vi "Calibration_CreateFromMatrix.vi"(1 "sample points":cluster{dbl, dbl}[](array[cluster])=[{0.0, 0.0}, {1.0, 0.0}, {0.0, 1.0}], 2 "Linear conversion Matrix":dbl[][](array[numeric])=[[1.0, 0.0, 0.0], [0.0, 1.0, 0.0]]) -> (0 "CalibrationCoordinates: x,x',y,y'...":dbl[][](array[numeric])=[[0.0, 0.0, 0.0, 0.0], [1.0, 1.0, 0.0, 0.0], [0.0, 0.0, 1.0, 1.0]])   [LabVIEW 2011]
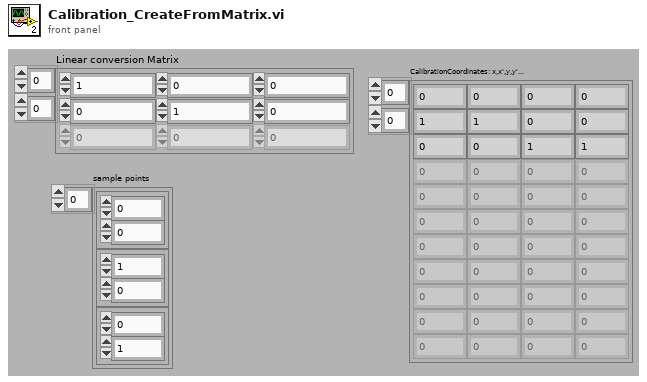
[diagram p1: front panel]
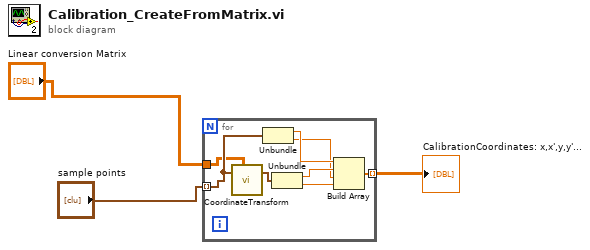
[diagram p0: block diagram]
diagram:
  n1 = for {
    tunnel: "Linear conversion Matrix" -> [w4]
    tunnel: "sample points" -> [w6] mode=indexing
    tunnel: [w11] -> w2 mode=indexing
    n2 = call "CoordinateTransform.vi"("input coordiantes"=w6, "Conversion Matrix"=w4) -> ("output coordiantes"=w5:cluster{"x":dbl, "y":dbl})  [unwired: 2 in, 1 out]
    n3 = Unbundle(w6) -> (w10:dbl, w8:dbl)
    n4 = Unbundle(w5) -> ("x"=w9:dbl, "y"=w7:dbl)
    n5 = Build Array(w10, w9, w8, w7) -> (w11:dbl[])
  }
  "CalibrationCoordinates: x,x',y,y'..." <- w2
